vi "Read AV Measurement.vi"(0 "VISA resource name":refnum<visa-resource-name>, 11 "error in (no error)":errorcluster) -> (4 "VISA resource name out":refnum<visa-resource-name>, 6 "AV Measurement Results":cluster{dbl[], dbl[]}(graph), 15 "error out":errorcluster)   [LabVIEW 2020, in "Keithley 648X Series.lvlib"]
doc: "Initiates the instrument and reads the fresh AV measurement readings.\n\n<b>Notes:</b>\n1)The <b>Arm AV Measurement</b> action VI must be used before this VI to activate the AV functionality.\n2) This is valid for <b>Model 6487 only</b>"
uses:
  <instrlib>/Keithley 648X Series/Keithley 648X Series.lvlib
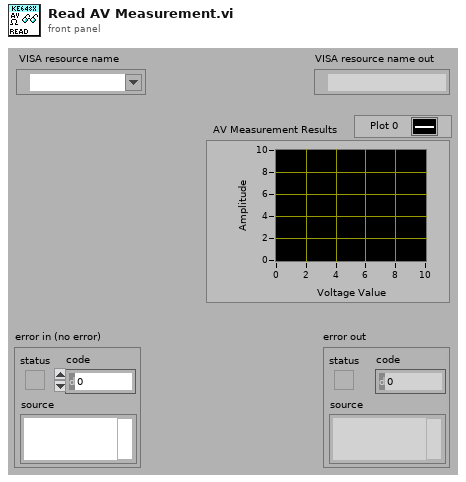
[diagram p1: front panel]
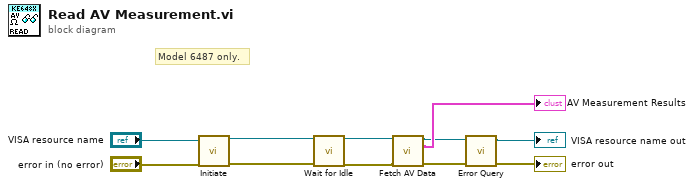
[diagram p0: block diagram]
diagram:
  # "Model 6487 only."
  n1 = call <instrlib>:"Initiate.vi"("VISA resource name"="VISA resource name", "error in (no error)"="error in (no error)") -> ("VISA resource name out"=w6:refnum<visa-resource-name>, "error out"=w7:errorcluster)  [unwired: 12 in]
  n2 = call <instrlib>:"Wait for Idle.vi"("VISA resource name"=w6, "error in (no error)"=w7) -> ("VISA resource name out"=w3:refnum<visa-resource-name>, "error out"=w4:errorcluster)  [unwired: 12 in]
  n3 = call <instrlib>:"Fetch AV Data.vi"("VISA resource name"=w3, "error in (no error)"=w4) -> ("VISA resource name out"=w1:refnum<visa-resource-name>, "AV Data"=→"AV Measurement Results":cluster{dbl[], dbl[]}, "error out"=w5:errorcluster)  [unwired: 11 in]
  n4 = call <instrlib>:"Error Query.vi"("error in (no error)"=w5, "VISA resource name"=w1) -> ("error out"=→"error out":errorcluster, "VISA resource name out"=→"VISA resource name out":refnum<visa-resource-name>)  [unwired: 6 in, 2 out]
